vi "Update Plugin to Abort.vi"(8 "error in (no error)":errorcluster, 11 "CIF_UI in":refnum<class "CIF_UI.lvclass">) -> (0 "error out":errorcluster, 3 "CIF_UI out":refnum<class "CIF_UI.lvclass">)   [LabVIEW 2021, in "CIF_UI.lvclass"]
uses:
  CIF_UI.lvclass
  CIF_UI.lvclass/CIF_UI.ctl
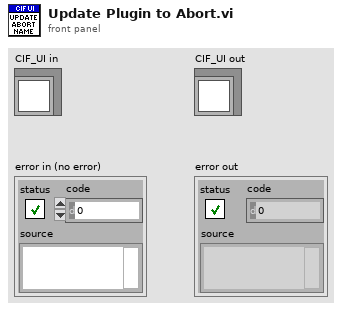
[diagram p1: front panel]
types:
  T1 = typedef "CIF_UI.lvclass/Plugin Connection Map.ctl" = map{string, T2}
  T2 = typedef "CIF_UI.lvclass/Plugin Connections.ctl" = cluster{"gRPC ID":T3, "Plugin Info":T4}
  T3 = typedef "grpc-lvsupport-release.lvlib/grpcId.ctl" = u64
  T4 = typedef "CIF_UI.lvclass/PluginInfo.ctl" = cluster{"Name":string, "Type":string, "grpc_port":i32, "Version":T5, "Node Status":T6}
  T5 = typedef "CIF_UI.lvclass/Version.ctl" = cluster{"Major":i32, "Minor":i32, "Fix":i32}
  T6 = typedef "CIFCoreCommon.lvlib/gRPC Reported Plugin Status.ctl" = cluster{"State":T7, "Timing Statistics (us)":T8, "FIFO Statistics (us)":T10, "error":T11, "Monitor Doubles":T12, "Monitor U64":T13, "Monitor I64":T14}
  T7 = typedef "CIFCoreCommon.lvlib/Plugin State.ctl" = enum32{"Null", "Creating", "Listening", "Running", "CleaningUp", "Destroying"}
  T8 = typedef "CIFCoreCommon.lvlib/Timing Statistics.ctl" = cluster{"Period":T9, "Wake Error":T9, "Execute":T9, "Housekeep":T9, "Idle":T9, "Cleanup":T9, "Custom 1 (custom units)":T9, "Custom 2 (custom units)":T9}
  T9 = typedef "CIFCoreCommon.lvlib/Timing Stats Base.ctl" = cluster{"Max":i64, "Avg":dbl, "Min":i64}
  T10 = typedef "CIFCoreCommon.lvlib/FIFO Statistics.ctl" = cluster{"From T0":T9, "From Previous Plugin":T9, "Output Error":T9}
  T11 = typedef "CIFCoreCommon.lvlib/Simple Error.ctl" = cluster{"status":bool, "code":i32}
  T12 = typedef "CIFCoreCommon.lvlib/Monitor Doubles.ctl" = cluster{"1":dbl, "2":dbl, "3":dbl, "4":dbl}
  T13 = typedef "CIFCoreCommon.lvlib/Monitor U64.ctl" = cluster{"1":u64, "2":u64, "3":u64, "4":u64}
  T14 = typedef "CIFCoreCommon.lvlib/Monitor I64.ctl" = cluster{"1":i64, "2":i64, "3":i64, "4":i64}
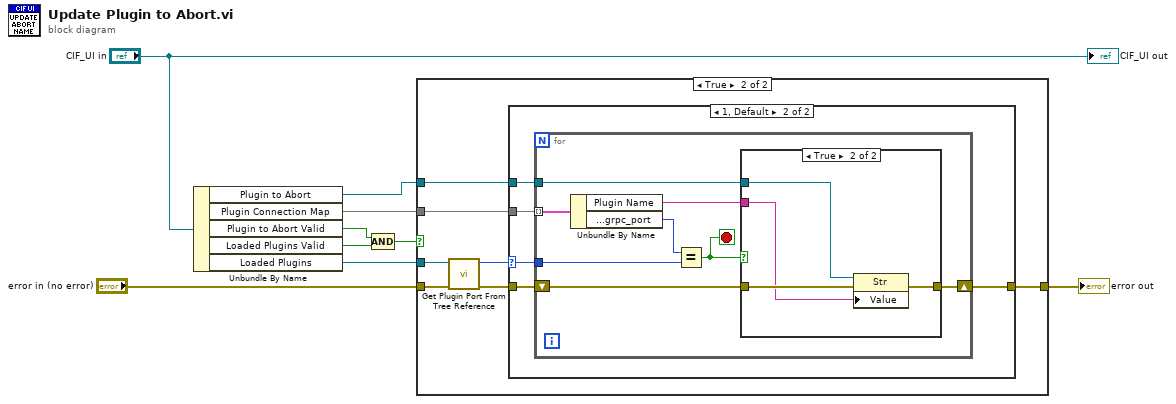
[diagram p0: block diagram]
diagram:
  n1 = Unbundle By Name("CIF_UI in") -> ("Plugin to Abort"=w1:refnum<vi>, "Plugin Connection Map"=w6:T1, "Plugin to Abort Valid"=w2:bool, "Loaded Plugins Valid"=w3:bool, "Loaded Plugins"=w9:refnum<vi>)
  n2 = Compound Arithmetic op=AND(w2, w3) -> (w8:bool)
  n3 = case shown="True" w8 {
    tunnel: w6 -> [_ w17]
    tunnel: "error in (no error)" -> [w10 w16]
    tunnel: w1 -> [_ w15]
    tunnel: w9 -> [_ w14]
    tunnel: [w10 w11] -> w7
    frame False {
    }
    frame True {
      n4 = call "Get Plugin Port From Tree Reference.vi"("error in (no error)"=w16, "Loaded Plugins"=w14) -> ("error out"=w13:errorcluster, "Plugin port"=w12:i32)  [unwired: 8 in]
      n5 = case shown="1, Default" w12 {
        selector: w12 -> [_ w20]
        tunnel: w17 -> [_ w23]
        tunnel: w15 -> [_ w22]
        tunnel: w13 -> [w18 w21]
        tunnel: [w18 w19] -> w11
        frame 0 {
        }
        frame 1, Default {
          n6 = for {
            tunnel: w23 -> [w31] mode=indexing
            tunnel: w20 -> [w30]
            tunnel: w22 -> [w26]
            shift-right: [w24] -> w19
            shift-left: w21 -> [w25]
            stop <- w28 stop-if-true
            n7 = Unbundle By Name(w31) -> ("Plugin Name"=w27:string, "Plugin Connections.Plugin Info.grpc_port"=w29:i32)
            n8 = Equal?(x=w29, y=w30) -> (x = y?=w28:bool)
            n9 = case shown="True" w28 {
              tunnel: w27 -> [_ w34]
              tunnel: w26 -> [_ w35]
              tunnel: w25 -> [w32 w36]
              tunnel: [w32 w33] -> w24
              frame False {
              }
              frame True {
                n10 = property class="Str"(reference=w35, error in=w36, "Value"=w34) -> (error out=w33:errorcluster)  [unwired: 1 out]
              }
            }
          }
        }
      }
    }
  }
  "error out" <- w7
  "CIF_UI out" <- "CIF_UI in"
